vi "Init Device.vi"(7 "Layout Ref":refnum<vi>, 8 "error in (no error)":errorcluster, 10 "Chan# Array":i32[](array[numeric]), 11 "Slave_Pulseblaster in":refnum<class "Slave_Pulseblaster.lvclass">) -> (0 "error out":errorcluster, 3 "Slave_Pulseblaster out":refnum<class "Slave_Pulseblaster.lvclass">)   [LabVIEW 2013, in "Slave_Pulseblaster.lvclass"]
doc: "Initialize the correct columns and their default appearance.\nUse the front panel to change default appearance of the device in the Add/Manage devices.\n\nOpen a specific device implementation for details."
uses:
  Slave_Pulseblaster.lvclass
  ColumnVIs/DigitalCol/DigitalCol.lvclass
  TypeDefs/DigitalColumnAppearCluster.ctl
  Slave_Pulseblaster.lvclass/Slave_Pulseblaster.ctl
  ColumnVIs/Column/Column.lvclass
panel:
  in  "Digital Column Defaults":T1={"Column Name"="", "Width"=15, "Bkgd"=[1985280, 6618880, 14090026], "Text"=[16448250, 0, 0]}
  in  "Board Number":i32=1 max=256 step=1
  in  "SpinAPI Path":path=path "C:/SpinCore/SpinAPI/dll/spinapi.dll"
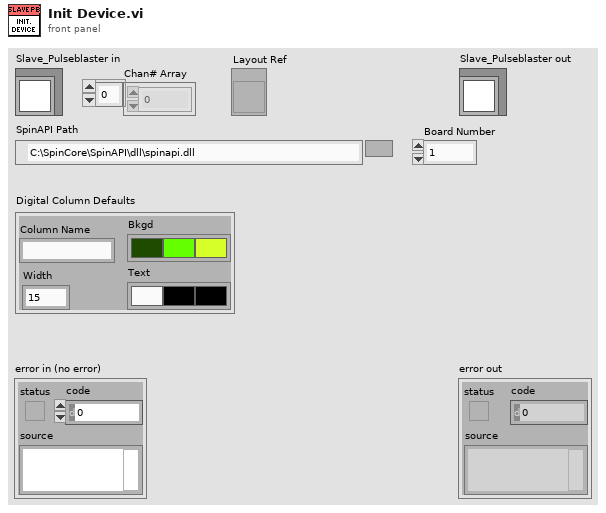
[diagram p1: front panel]
types:
  T1 = typedef "DigitalColumnAppearCluster.ctl" = cluster{"Column Name":string, "Width":u32, "Bkgd":u32[], "Text":u32[]}
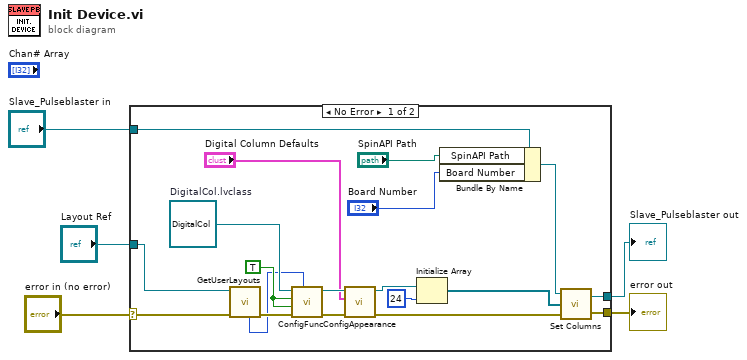
[diagram p0: block diagram]
diagram:
  n1 = case shown="No Error" "error in (no error)" {
    selector: "error in (no error)" -> [w11 w25]
    tunnel: "Slave_Pulseblaster in" -> [w23 w26]
    tunnel: [w7 w26] -> w4
    tunnel: [w6 w25] -> w3
    tunnel: "Layout Ref" -> [w14 _]
    frame No Error {
      w19 = TRUE ("Disableable? (True)")
      w20 = refnum<class "DigitalCol.lvclass"> refnum  # DigitalCol.lvclass
      n2 = call "GetUserLayouts.vi"("error in (no error)"=w11, "Layout Ring Refnum"=w14) -> ("error out"=w13:errorcluster, "Num User Layouts"=w12:i32)  [unwired: 5 in, 3 out]
      n3 = call "ConfigFunc.vi"("Num Layouts (ignored)"=w12, "error in (no error)"=w13, "isVariable? (True)"=w19, "Disableable? (True)"=w19, "Column in"=w20) -> ("error out"=w18:errorcluster, "Column out"=w17:refnum<class "DigitalCol.lvclass">)  [unwired: 5 in]
      n4 = call "ConfigAppearance.vi"("error in (no error)"=w18, "Column Appearance"="Digital Column Defaults", "Column in"=w17) -> ("error out"=w8:errorcluster, "Column out"=w15:refnum<class "DigitalCol.lvclass">)  [unwired: 7 in]
      n5 = Initialize Array(w15, 24 ("dimension size")) -> (w10:refnum<class "DigitalCol.lvclass">[])
      n6 = Bundle By Name(cluster=w23, "SpinAPI Path"="SpinAPI Path", "Board Number"="Board Number") -> (w9:refnum<class "Slave_Pulseblaster.lvclass">)
      n7 = call-dynamic "Set Columns.vi"("error in (no error)"=w8, "Columns in"=w10, "Pulseblaster in"=w9) -> ("error out"=w6:errorcluster, "Pulseblaster out"=w7:refnum<class "Slave_Pulseblaster.lvclass">)  [unwired: 1 in]
    }
    frame Error {
    }
  }
  "error out" <- w3
  "Slave_Pulseblaster out" <- w4
